vi "Ejercicio practica.vi"() -> ()   [LabVIEW 2011]
panel:
  out "Temp Mayor":dbl
  out "Temp Promedio":dbl
  out "61-100":bool
  out "31-60":bool
  out "1-30":bool
  out "Temperatura":dbl(slide) scale=0.0..100.0
  # "Generar la temperatura entre 1-100 el\nprograma se detiene cuando la temperatura\nes mayor a 90.\nAl final debera presentar la temp promedio.\nDurante el programa se ejecute debera de\nencender los led de acuerdo al rango.\nObtener la temp mayor."
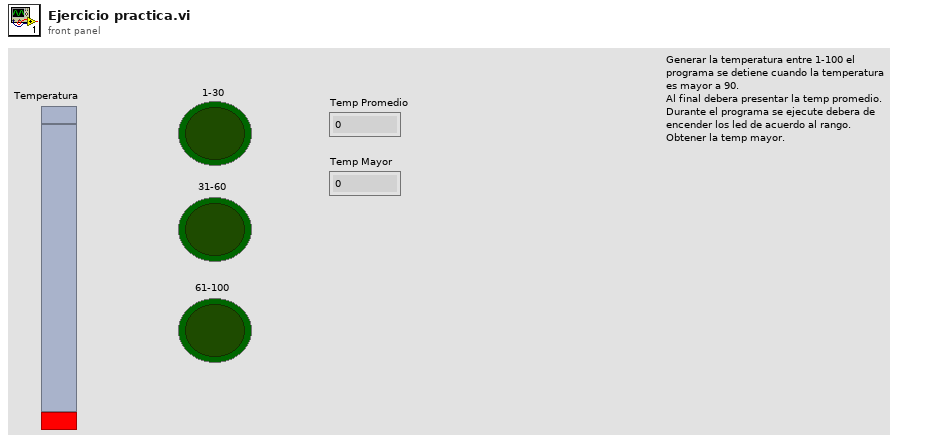
[diagram p1: front panel]
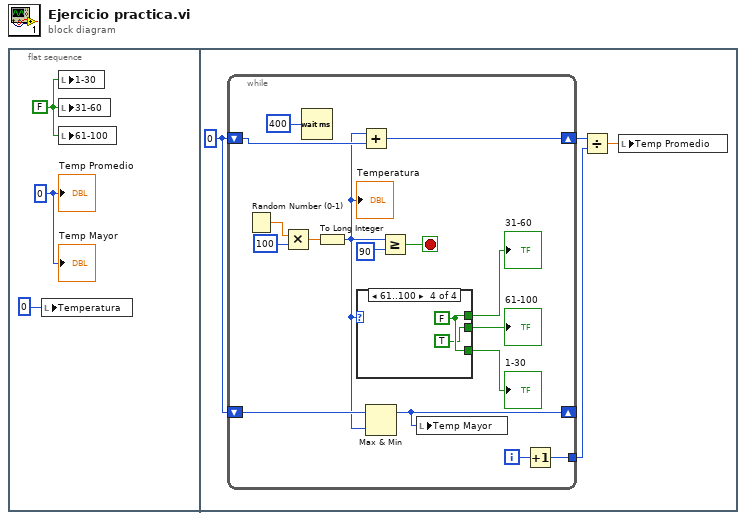
[diagram p0: block diagram]
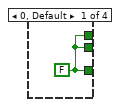
[diagram p2: hidden frame]
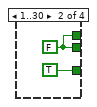
[diagram p3: hidden frame]
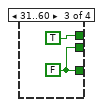
[diagram p4: hidden frame]
diagram:
  n1 = flat-sequence {
    frame #0 {
      w1 = 0
      w2 = FALSE
      n2 = local write "Temperatura"(0) -> ()
      n3 = local write "1-30"(w2) -> ()
      n4 = local write "31-60"(w2) -> ()
      n5 = local write "61-100"(w2) -> ()
      "Temp Promedio" <- w1
      "Temp Mayor" <- w1
    }
    frame #1 {
      w7 = 0
      n6 = while {
        shift-right: [w12] -> _
        shift-left: w7 -> [w13]
        shift-right: [w19] -> w4
        shift-left: w7 -> [w20]
        tunnel: [w14] -> w5
        i -> [w15]
        stop <- w11 stop-if-true
        n7 = Random Number (0-1)() -> (number: 0 to 1=w23:dbl)
        n8 = Multiply(x=w23, y=100) -> (x*y=w21:dbl)
        n9 = Wait (ms)(milliseconds to wait=400) -> ()  [unwired: 1 out]
        n10 = To Long Integer(number=w21) -> (32bit integer=w9:i32)
        "Temperatura" <- w9
        n11 = case shown="61..100" w9 {
          tunnel: [w24 TRUE w27 w30] -> w18
          tunnel: [w24 w25 TRUE w30] -> w17
          tunnel: [w24 w25 w27 TRUE] -> w16
          frame 0, Default {
            w24 = FALSE
          }
          frame 1..30 {
            w25 = FALSE
          }
          frame 31..60 {
            w27 = FALSE
          }
          frame 61..100 {
            w30 = FALSE
          }
        }
        "1-30" <- w18
        "31-60" <- w17
        "61-100" <- w16
        n12 = Add(x=w9, y=w20) -> (x+y=w19:i32)
        n13 = Max & Min(x=w13, y=w9) -> (max(x,y)=w12:i32)  [unwired: 1 out]
        n14 = Greater Or Equal?(x=w9, y=90) -> (x >= y?=w11:bool)
        n15 = local write "Temp Mayor"(w12) -> ()
        n16 = Increment(x=w15) -> (x+1=w14:i32)
      }
      n17 = Divide(x=w4, y=w5) -> (x/y=w6:dbl)
      n18 = local write "Temp Promedio"(w6) -> ()
    }
  }
